vi "convertAnalogData.vi"(8 "error in (no error)":errorcluster, 10 "Data":T1={"Timestamps ms"=[0.0, 0.005, 0.009, 0.012], "DataPerChannel"=[]} {"Timestamps ms" format="%.3f"}, 11 "DIO64Output in":refnum<class "DIO64Output.lvclass">) -> (0 "error out":errorcluster, 2 "digitalData":T2={"Timestamps ms"=[0.0, 0.005, 0.009, 0.012], "Bitmap"=[[TRUE, FALSE, FALSE, FALSE, FALSE, FALSE, FALSE, FALSE, FALSE, TRUE, TRUE, FALSE, FALSE, FALSE, FALSE, FALSE], [FALSE, FALSE, FALSE, FALSE, FALSE, FALSE, FALSE, FALSE, FALSE, FALSE, FALSE, FALSE, FALSE, FALSE, FALSE, TRUE], [FALSE, FALSE, FALSE, FALSE, TRUE, FALSE, FALSE, FALSE, FALSE, FALSE, FALSE, FALSE, FALSE, FALSE, FALSE, FALSE]]} {"Timestamps ms" format="%.3f"}, 3 "DIO64Output out":refnum<class "DIO64Output.lvclass">)   [LabVIEW 2011, in "Hardware.lvlib" / "Channels.lvlib" / "DIO64Output.lvclass"]
uses:
  DIO64Output.lvclass
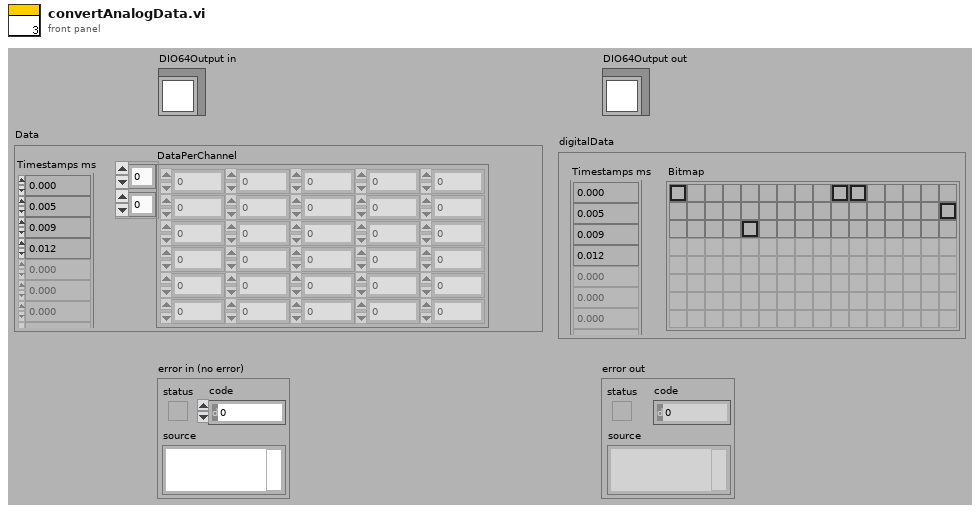
[diagram p1: front panel]
types:
  T1 = cluster{"Timestamps ms":dbl[], "DataPerChannel":dbl[][]}
  T2 = cluster{"Timestamps ms":dbl[], "Bitmap":bool[][]}
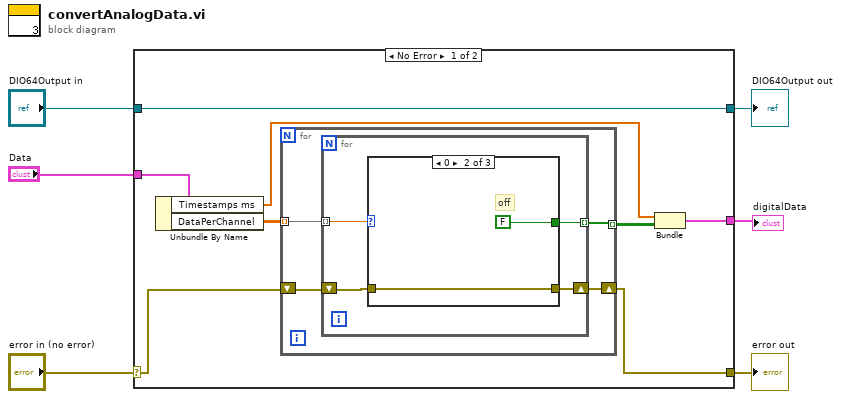
[diagram p0: block diagram]
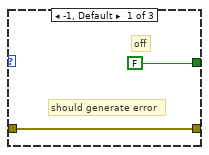
[diagram p2: hidden frame]
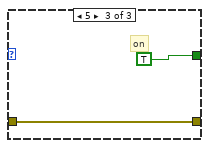
[diagram p3: hidden frame]
diagram:
  n1 = case shown="No Error" "error in (no error)" {
    selector: "error in (no error)" -> [w11 w30]
    tunnel: [w7 w30] -> w5
    tunnel: [w14 w29] -> w3
    tunnel: "DIO64Output in" -> [w14 w29]
    tunnel: "Data" -> [w13 _]
    tunnel: [w8 _] -> w1
    frame No Error {
      n2 = Unbundle By Name(w13) -> ("Timestamps ms"=w10:dbl[], "DataPerChannel"=w12:dbl[][])
      n3 = for {
        tunnel: w12 -> [w18] mode=indexing
        shift-right: [w16] -> w7
        shift-left: w11 -> [w17]
        tunnel: [w15] -> w9 mode=indexing
        n4 = for {
          tunnel: w18 -> [w22] mode=indexing
          shift-right: [w20] -> w16
          shift-left: w17 -> [w21]
          tunnel: [w19] -> w15 mode=indexing
          n5 = case shown="0" w22 {
            tunnel: [FALSE FALSE TRUE] -> w19
            tunnel: w21 -> [w23 w25 w27]
            tunnel: [w23 w25 w27] -> w20
            frame -1, Default {
              # "should generate error"
              # "off"
            }
            frame 0 {
              # "off"
            }
            frame 5 {
              # "on"
            }
          }
        }
      }
      n6 = Bundle("Timestamps ms"=w10, w9) -> (w8:cluster{"Timestamps ms":dbl[], bool[][]})  [unwired: 1 in]
    }
    frame Error {
    }
  }
  "error out" <- w5
  "DIO64Output out" <- w3
  "digitalData" <- w1
